vi "Scan Calculations.vi"(0 "counter cluster in":T9, 1 "control flags in":T8, 2 "bleach mode":bool, 3 "N spot tracker in":T5, 4 "scan specification in":T10={"z resolution (pixels)"=1000, "iterations per pixel"=28, "iterations per z-scan (=zres*iterperpixel)"=50, "x resolution (pixels)"=100, "y resolution (pixels)"=80, "number of z-lines per volume"=30, "number of repetitions (volumes)"=5, "Pockels cell voltage (bits)"=-1, "Vx center (bits)"=0, "Vy center (bits)"=0, "Vx amplitude (bits)"=40, "Vy amplitude (bits)"=0, "lines to delay between scan start and output"=1, "LSB has acquire control"=FALSE, "Pockels cell bleach voltage"=0}, 5 "tracking settings":T12, 6 "ff vel?":bool, 7 "3-axis PV tracking state in":T6, 8 "x-y phase shift (*2^16/2*pi)":u16=16384, 9 "min photons for update":u32=30, 10 "reset flags":u8, 11 "spot location constraints":T2=[{"spot number"=0, "active"=FALSE, "x max"=0, "x min"=0, "y max"=0, "y min"=0}, {"spot number"=0, "active"=FALSE, "x max"=0, "x min"=0, "y max"=0, "y min"=0}, {"spot number"=0, "active"=FALSE, "x max"=0, "x min"=0, "y max"=0, "y min"=0}, {"spot number"=0, "active"=FALSE, "x max"=0, "x min"=0, "y max"=0, "y min"=0}], 12 "pockels always on":bool, 13 "current location":T4, 15 "stim duration":u16=20, 18 "stim by cycle settings":T1={"stim by cycle"=FALSE, "stim enable"=FALSE, "lines per stim"=42, "total cycles per stim cycle"=10}, 19 "stim delay":i16=5) -> (14 "end scan":bool, 16 "trigger out":bool, 17 "kalman to host":cluster{"Kalman State":T7, "Kalman Update":bool}, 20 "counter cluster out":T9, 21 "control flags out":T8, 23 "N spot tracker out":T5, 24 "scan specification out":T10, 25 "DAC voltages":T11 {"pockels" max=4095 step=1; "y" max=4095 step=1; "x" max=4095 step=1}, 27 "3-axis PV tracking state out":T6={"x state"={"pos estimate"=0.0, "v estimate"=0.0, "weighted position error sum"=0.0, "photon count"=0, "transmit tick count"=0, "axis number"=0, "px (levels^2)"=0.0, "pxv (levels^2/ticks)"=0.0, "pv (levels^2/ticks^2)"=0.0, "vel diff (levels^2/ticks^3)"=0.0, "gx"=0.0, "rtwiddle"=0.0, "photon count ch0"=0, "photon count ch1"=0, "Dx -levels^2/ticks"=0.0}, "y state"={"pos estimate"=0.0, "v estimate"=0.0, "weighted position error sum"=0.0, "photon count"=0, "transmit tick count"=0, "axis number"=1, "px (levels^2)"=0.0, "pxv (levels^2/ticks)"=0.0, "pv (levels^2/ticks^2)"=0.0, "vel diff (levels^2/ticks^3)"=0.0, "gx"=0.0, "rtwiddle"=0.0, "photon count ch0"=0, "photon count ch1"=0, "Dx -levels^2/ticks"=0.0}, "z state"={"pos estimate"=0.0, "v estimate"=0.0, "weighted position error sum"=0.0, "photon count"=0, "transmit tick count"=0, "axis number"=2, "px (levels^2)"=0.0, "pxv (levels^2/ticks)"=0.0, "pv (levels^2/ticks^2)"=0.0, "vel diff (levels^2/ticks^3)"=0.0, "gx"=0.0, "rtwiddle"=0.0, "photon count ch0"=0, "photon count ch1"=0, "Dx -levels^2/ticks"=0.0}, "spot number"=0})   [LabVIEW 2010]
uses:
  FPGA tracking/polar tracking settings.ctl
  common_typedefs/DAC_voltage_tagResonantr.ctl
  scan_specification_tagResonant.ctl
  counter_cluster_tagResonant.ctl
  FPGA tracking/kalman 3-axis state.ctl
  FPGA tracking/integrating single axis kalman state.ctl
  FPGA tracking/control flags.ctl
  FPGA tracking/kalman N spot state.ctl
  FPGA tracking/spot location constraints.ctl
  FPGA tracking/spot location constraint.ctl
  <vilib>/eio/EIONode/EIONode.xnode
  <vilib>/rvi/eio/nirviEIOImplementation/nirviEIOImplementation.xnode
  <vilib>/rvi/eio/common/nirviEmuClasses.ctl
  <vilib>/rvi/eio/common/nirviEmuTemplateMethod_noerrors.vi
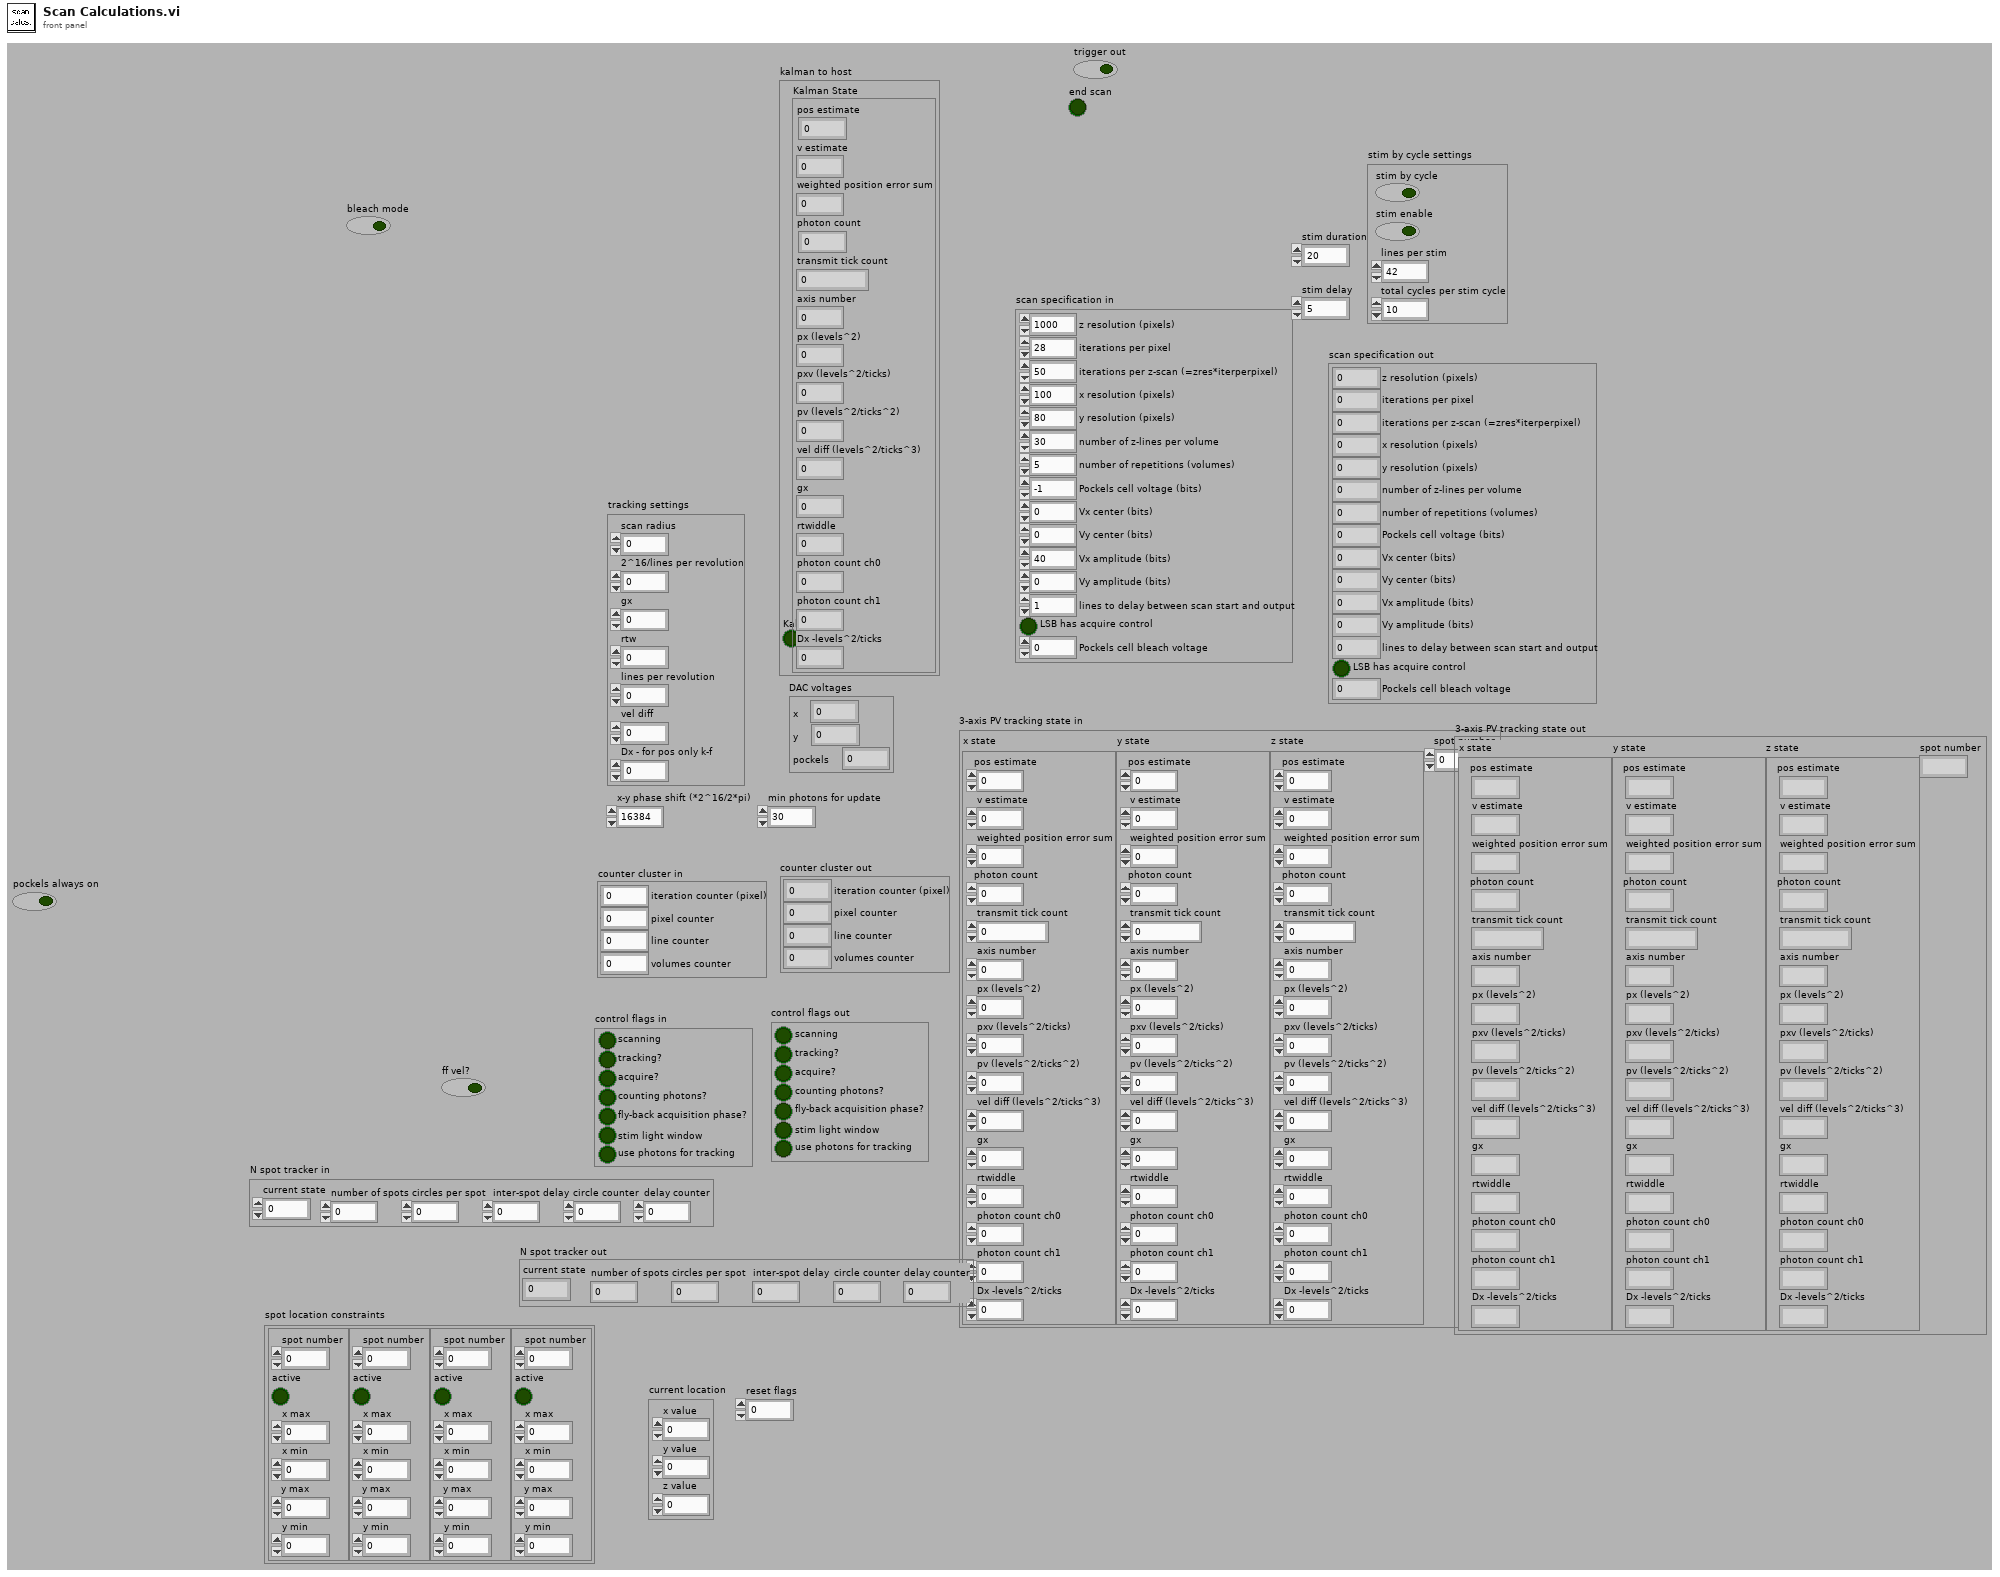
[diagram p1: front panel]
types:
  T1 = cluster{"stim by cycle":bool, "stim enable":bool, "lines per stim":u16, "total cycles per stim cycle":u16}
  T2 = typedef "spot location constraints.ctl" = T3[]
  T3 = typedef "spot location constraint.ctl" = cluster{"spot number":i8, "active":bool, "x max":i16, "x min":i16, "y max":i16, "y min":i16}
  T4 = cluster{"x value":i16, "y value":i16, "z value":i16}
  T5 = typedef "kalman N spot state.ctl" = cluster{"current state":u8, "number of spots":u8, "circles per spot":u16, "inter-spot delay":u8, "circle counter":u16, "delay counter":u8}
  T6 = typedef "kalman 3-axis state.ctl" = cluster{"x state":T7, "y state":T7, "z state":T7, "spot number":u8}
  T7 = typedef "integrating single axis kalman state.ctl" = cluster{"pos estimate":fxp<+/-,32,16>, "v estimate":fxp<+/-,16,0>, "weighted position error sum":fxp<+/-,32,32>, "photon count":u32, "transmit tick count":u32, "axis number":u8, "px (levels^2)":fxp<+,32,19>, "pxv (levels^2/ticks)":fxp<+,32,2>, "pv (levels^2/ticks^2)":fxp<+,32,-14>, "vel diff (levels^2/ticks^3)":fxp<+,24,-22>, "gx":fxp<+,16,8>, "rtwiddle":fxp<+,16,26>, "photon count ch0":u32, "photon count ch1":u32, "Dx -levels^2/ticks":fxp<+,32,19>}
  T8 = typedef "control flags.ctl" = cluster{"scanning":bool, "tracking?":bool, "acquire?":bool, "counting photons?":bool, "fly-back acquisition phase?":bool, "stim light window":bool, "use photons for tracking":bool}
  T9 = typedef "counter_cluster_tagResonant.ctl" = cluster{"iteration counter (pixel)":u16, "pixel counter":u16, "line counter":i16, "volumes counter":u16}
  T10 = typedef "scan_specification_tagResonant.ctl" = cluster{"z resolution (pixels)":u16, "iterations per pixel":u16, "iterations per z-scan (=zres*iterperpixel)":u16, "x resolution (pixels)":u16, "y resolution (pixels)":u16, "number of z-lines per volume":u16, "number of repetitions (volumes)":i32, "Pockels cell voltage (bits)":i16, "Vx center (bits)":i16, "Vy center (bits)":i16, "Vx amplitude (bits)":i16, "Vy amplitude (bits)":i16, "lines to delay between scan start and output":u16, "LSB has acquire control":bool, "Pockels cell bleach voltage":i16}
  T11 = typedef "DAC_voltage_tagResonantr.ctl" = cluster{"x":i16, "y":i16, "pockels":i16}
  T12 = typedef "polar tracking settings.ctl" = cluster{"scan radius":u16, "2^16/lines per revolution":u16, "gx":fxp<+,16,8>, "rtw":fxp<+,16,26>, "lines per revolution":u8, "vel diff":fxp<+,24,-22>, "Dx - for pos only k-f":fxp<+,32,19>}
  T13 = cluster{"update x":bool, "update y":bool, "update z":bool}
  T14 = cluster{"counts per cycle":u16, "num triggers":u32, "fb end":u16, "fb start":u16, "ff start":u16, "ff end":u16}
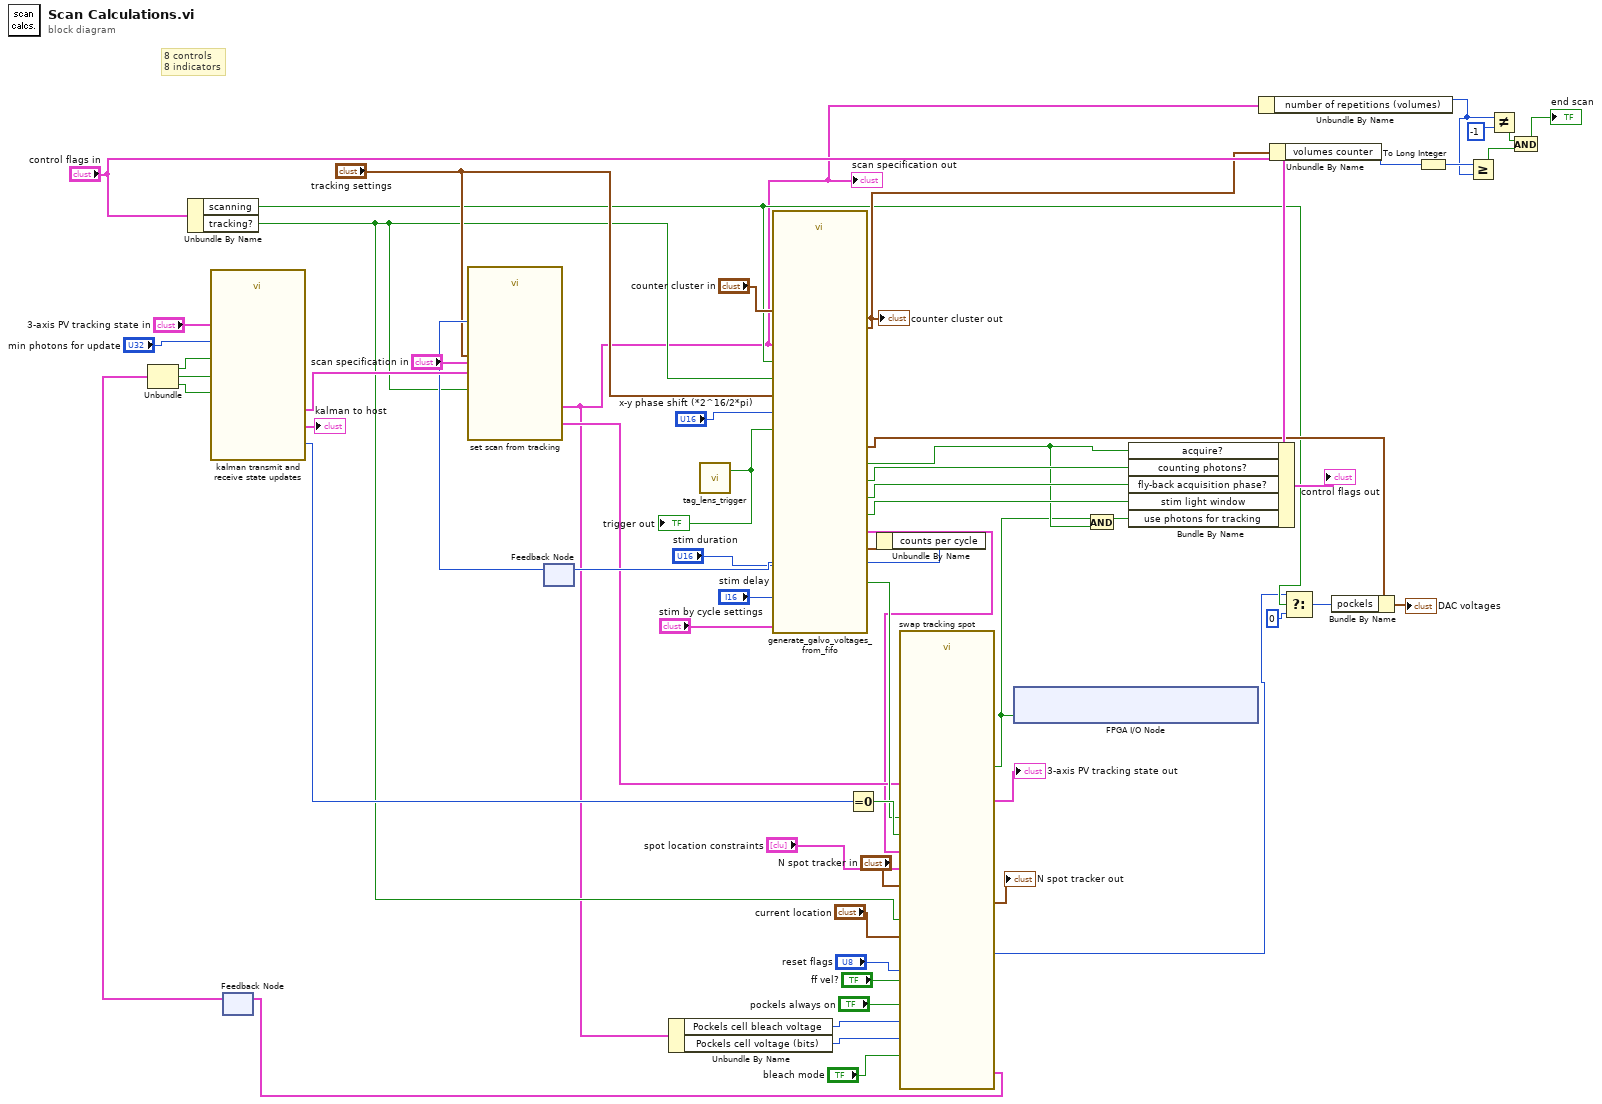
[diagram p0: block diagram]
diagram:
  # "8 controls\n8 indicators"
  n1 = Unbundle By Name("control flags in") -> ("scanning"=w8:bool, "tracking?"=w10:bool)
  n2 = feedback #1() -> (w22:T13)  [unwired: 1 in]
  n3 = Unbundle(w22) -> ("update x"=w52:bool, "update y"=w51:bool, "update z"=w50:bool)
  n4 = call "kalman transmit and receive state updates.vi"("min photons to update"="min photons for update", "update z"=w50, "update y"=w51, "update x"=w52, "3-axis PV tracking state"="3-axis PV tracking state in") -> ("num kalmans queued"=w25:u16, "3-axis PV tracking state out"=w60:T6, "kalman to host"=→"kalman to host":cluster{"Kalman State":T7, "Kalman Update":bool})  [unwired: 3 in, 1 out]
  n5 = feedback #2() -> (w53:u16)  [unwired: 1 in]
  n6 = call "set scan from tracking.vi"("tracking?"=w10, "counts per cycle"=w53, "tracking settings"="tracking settings", "tracking state in"=w60, "scan specification"="scan specification in") -> ("tracking state out"=w27:T6, "scan specification out"=w6:T10)  [unwired: 5 in]
  "scan specification out" <- w6
  n7 = Unbundle By Name(w6) -> ("Pockels cell bleach voltage"=w5:i16, "Pockels cell voltage (bits)"=w4:i16)
  n8 = call "tag_lens_trigger.vi"() -> ("trigger out"=w57:bool)  [unwired: 2 in]
  "trigger out" <- w57
  n9 = call "generate_galvo_voltages_from_fifo.vi"("resonant trigger"=w57, "counter cluster in"="counter cluster in", "stim duration"="stim duration", "tracking settings"="tracking settings", "scan specification"=w6, "scanning"=w8, "tracking"=w10, "x-y phase shift (*2^16/2*pi)"="x-y phase shift (*2^16/2*pi)", "stim by cycle settings"="stim by cycle settings", "stim delay"="stim delay") -> ("stim light window"=w45:bool, "trigger diagnostics"=w55:T14, "update tracking?"=w24:T13, "counting photons?"=w32:bool, "DAC voltages"=w15:T11, "counter cluster out"=w35:T9, "new circle"=w28:bool, "fly-back acquisition phase?"=w46:bool, "acquire?"=w17:bool)  [unwired: 1 in]
  "counter cluster out" <- w35
  n10 = Equal To 0?(x=w25) -> (x = 0?=w29:bool)
  n11 = Unbundle By Name(w55) -> ("counts per cycle"=w54:u16)
  n12 = feedback-in #2(w54) -> ()
  n13 = call "swap tracking spot.vi"("N spot tracker in"="N spot tracker in", "tracking state in"=w27, "bleach mode"="bleach mode", "reset flags"="reset flags", "new circle"=w28, "permission to swap states"=w29, "tracking?"=w10, "spot location constraints"="spot location constraints", "pockels normal"=w4, "pockels bleach"=w5, "current location"="current location", "update tracking? in"=w24, "pockels always on"="pockels always on", "ff vel?"="ff vel?") -> ("N spot tracker out"=→"N spot tracker out":T5, "tracking state out"=→"3-axis PV tracking state out":T6, "update tracking? out"=w23:T13, "pockels voltage"=w7:i16, "use photons to track"=w13:bool)  [unwired: 1 in]
  n14 = feedback-in #1(w23) -> ()
  n15 = xnode "FPGA I/O Node"("Connector0/DIO9 (feedback engaged)"=w13) -> ()  [unwired: 1 in, 1 out]
  n16 = And(x=w13, y=w17) -> (x .and. y?=w18:bool)
  n17 = Bundle By Name(cluster="control flags in", "acquire?"=w17, "counting photons?"=w32, "fly-back acquisition phase?"=w46, "stim light window"=w45, "use photons for tracking"=w18) -> (→"control flags out":T8)
  n18 = Unbundle By Name(w6) -> ("number of repetitions (volumes)"=w37:i32)
  n19 = Unbundle By Name(w35) -> ("volumes counter"=w39:u16)
  n20 = Select(t=w7, s=w8, f=i16 0) -> (s? t:f=w12:i16)
  n21 = Bundle By Name(cluster=w15, "pockels"=w12) -> (→"DAC voltages":T11)
  n22 = To Long Integer(number=w39) -> (32bit integer=w38:i32)
  n23 = Greater Or Equal?(x=w38, y=w37) -> (x >= y?=w41:bool)
  n24 = Not Equal?(x=w37, y=-1) -> (x != y?=w40:bool)
  n25 = And(x=w40, y=w41) -> (x .and. y?=→"end scan":bool)
